vi "GetPinFunctions.vi"(0 "VISA Refnum in":refnum<visa-resource-name>, 2 "Address":u8, 3 "error in (no error)":errorcluster) -> (1 "S3Mode":u8, 4 "S5Mode":u8, 5 "VISA Refnum out":refnum<visa-resource-name>, 6 "Valid":bool, 7 "S4Mode":u8, 8 "error out":errorcluster)   [LabVIEW 2015, in "Ion Motion Roboclaw.lvlib"]
uses:
  <instrlib>/Ion Motion Roboclaw/Ion Motion Roboclaw.lvlib
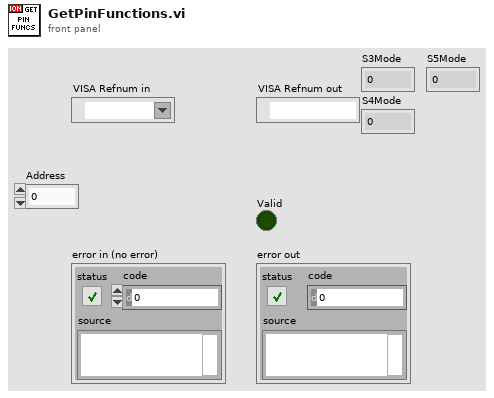
[diagram p1: front panel]
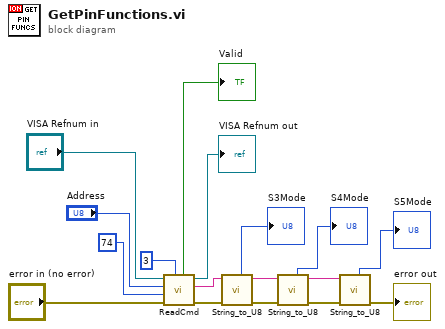
[diagram p0: block diagram]
diagram:
  n1 = call <instrlib>:"ReadCmd.vi"("Read Count"=u32 3, "error in (no error)"="error in (no error)", "Cmd"=u8 74, "Address"="Address", "VISA Refnum in"="VISA Refnum in") -> ("error out"=w9:errorcluster, "Output"=w8:string, "VISA Refnum out"=→"VISA Refnum out":refnum<visa-resource-name>, "Valid"=→"Valid":bool)  [unwired: 3 in]
  n2 = call <instrlib>:"String_to_U8.vi"("error in (no error)"=w9, "String"=w8) -> ("error out"=w15:errorcluster, "rest of the binary string"=w17:string, "Argument"=→"S3Mode":u8)  [unwired: 5 in]
  n3 = call <instrlib>:"String_to_U8.vi"("error in (no error)"=w15, "String"=w17) -> ("error out"=w14:errorcluster, "rest of the binary string"=w16:string, "Argument"=→"S4Mode":u8)  [unwired: 5 in]
  n4 = call <instrlib>:"String_to_U8.vi"("error in (no error)"=w14, "String"=w16) -> ("error out"=→"error out":errorcluster, "Argument"=→"S5Mode":u8)  [unwired: 5 in, 1 out]
